vi "PWM Pulsate (Session).vi"() -> ()   [LabVIEW 2020, in "CTI-Scratchpad.lvlib"]
uses:
  CTI-Scratchpad.lvlib
  CTI/GPIO Number.ctl
  CTI/Session/Session.lvclass
  <vilib>/ptbypt/NI_PtbyPt.lvlib
  CTI/VisaComms/VisaComms.lvclass
  CTI/CTI.lvlib
panel:
  in  "Speed":i32(slide) scale=1000.0..1.0
  in  "stop":bool
  out "Act. Duty":sgl format="%_6f"
  in  "Port":refnum<visa-resource-name>="COM3"
  in  "Channel":T1
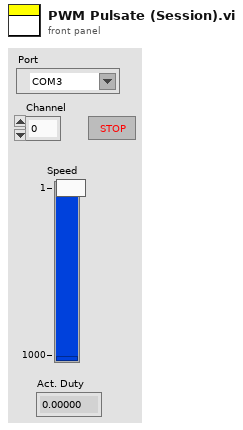
[diagram p1: front panel]
types:
  T1 = typedef "CTI.lvlib/GPIO Number.ctl" = i8
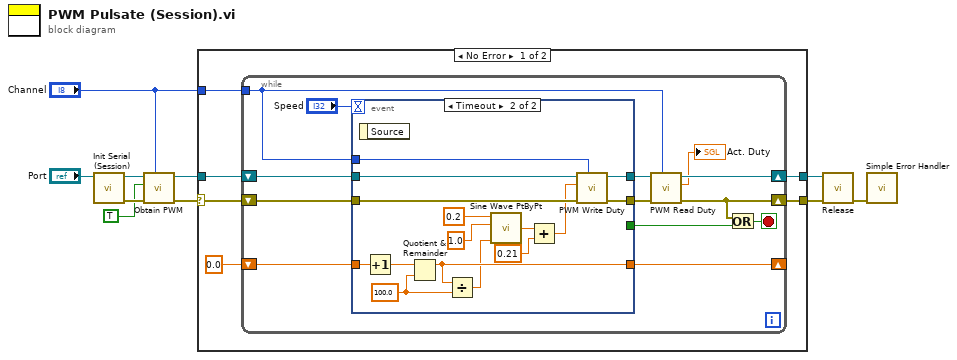
[diagram p0: block diagram]
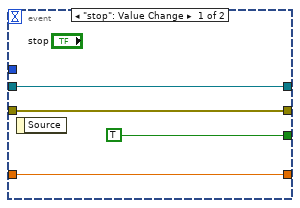
[diagram p2: hidden frame]
diagram:
  n1 = call "Init Serial (Session).vi"("VISA resource name in"="Port") -> ("error out"=w8:errorcluster, "Session"=w9:refnum<class "Session.lvclass">)  [unwired: 8 in, 1 out]
  n2 = call "Obtain PWM.vi"("GPIO #"="Channel", "error in (no error)"=w8, "Enable (F)"=TRUE, "Session in"=w9) -> ("error out"=w7:errorcluster, "Session out"=w6:refnum<class "Session.lvclass">)  [unwired: 6 in]
  n3 = case shown="No Error" w7 {
    selector: w7 -> [w15 w49]
    tunnel: w6 -> [w16 w50]
    tunnel: [w14 w50] -> w4
    tunnel: [w13 w49] -> w5
    tunnel: "Channel" -> [w12 _]
    frame No Error {
      n4 = while {
        shift-right: [w22] -> w14
        shift-left: w16 -> [w28]
        shift-right: [w21] -> w13
        shift-left: w15 -> [w27]
        tunnel: w12 -> [w18]
        shift-right: [w19] -> _
        shift-left: 0.0 -> [w20]
        stop <- w29 stop-if-true
        n5 = event shown="[1] Timeout" {
          selector: _ -> [_ _]
          dyn-events: _ -> [_ _]
          timeout: "Speed" -> [_ _]
          tunnel: [w33 w41] -> w25
          tunnel: w28 -> [w33 w46]
          tunnel: [w32 w42] -> w24
          tunnel: w27 -> [w32 w45]
          tunnel: [TRUE _] -> w26
          tunnel: w20 -> [w30 w40]
          tunnel: [w30 w37] -> w19
          tunnel: w18 -> [_ w35]
          event "stop": Value Change {
            n6 = event-data() -> ()  [unwired: 1 in, 1 out]
          }
          event Timeout {
            w38 = 100.0 ("frequency")
            n7 = event-data() -> ()  [unwired: 1 in, 1 out]
            n8 = Increment(x=w40) -> (x+1=w39:dbl)
            n9 = Quotient & Remainder(x=w39, y=w38) -> (x-y*floor(x/y)=w37:dbl)  [unwired: 1 out]
            n10 = Divide(x=w37, y=w38) -> (x/y=w36:dbl)
            n11 = call <vilib>:"Sine Wave PtByPt.vi"("time"=w36, "frequency"=1.0, "amplitude"=0.2) -> ("sine wave"=w44:dbl)  [unwired: 1 in]
            n12 = Add(x=w44, y=0.21) -> (x+y=w34:dbl)
            n13 = call "PWM Write Duty.vi"("GPIO #"=w35, "error in (no error)"=w45, "Duty % (0-1)"=w34, "Session in"=w46) -> ("error out"=w42:errorcluster, "Session out"=w41:refnum<class "Session.lvclass">)  [unwired: 6 in]
          }
        }
        n14 = call "PWM Read Duty.vi"("GPIO #"=w18, "error in (no error)"=w24, "Session in"=w25) -> ("error out"=w21:errorcluster, "Duty % (0-1)"=→"Act. Duty":sgl, "Session out"=w22:refnum<class "Session.lvclass">)  [unwired: 6 in]
        n15 = Or(x=w21, y=w26) -> (x .or. y?=w29:bool)
      }
    }
    frame Error {
    }
  }
  n16 = call-dynamic "Release.vi"("error in (no error)"=w5, "Session in"=w4) -> ("error out"=w3:errorcluster)  [unwired: 9 in]
  n17 = call <vilib>:"Simple Error Handler.vi"("error in (no error)"=w3) -> ()  [unwired: 4 in, 5 out]
